vi "GV stage as trigger.vi"() -> ()   [LabVIEW 2017]
panel:
  out "StageAsTrigger":bool
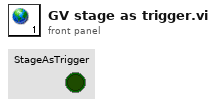
[diagram p1: front panel]
diagram:
